vi "Położenie robota z uwzględnieniem jego ewentualnej zmiany.vi"(6 "Boolean in":refnum<vi>, 7 "Parametry robota":T1={"Promień koła [m]"=0.045, "Szerokość robota [m]"=0.37}, 9 "Nowa Odl. od startu[m]":cluster{"X [m]":dbl, "Y [m]":dbl}={"X [m]"=-27.201483053257306, "Y [m]"=-30.40589390754667}, 10 "Azymut robota pocz./nowy":dbl, 11 "Prędkości kół":cluster{"prawe [rad/s]":dbl, "lewe [rad/s]":dbl}) -> (0 "Zmiana położenia robota?":bool, 1 "Azymut [stopnie]":dbl, 2 "Odległość robota od startu":cluster{"X[m]":dbl, "Y[m]":dbl})   [LabVIEW 2012, in "Biblioteka moduł map v3.lvlib" / "Matematyczne.lvlib"]
uses:
  Matematyczne.lvlib
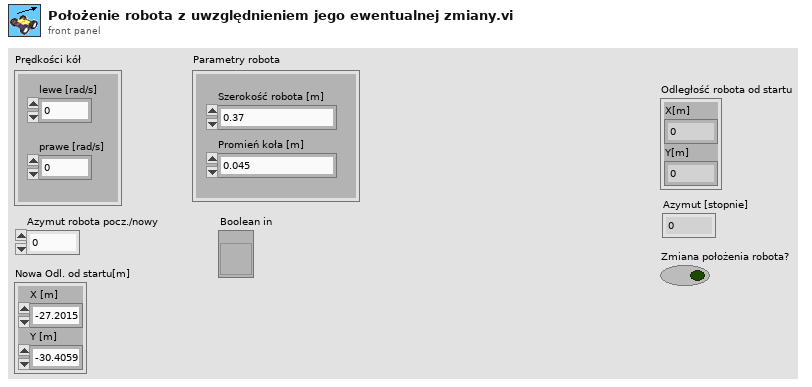
[diagram p1: front panel]
types:
  T1 = cluster{"Promień koła [m]":dbl, "Szerokość robota [m]":dbl}
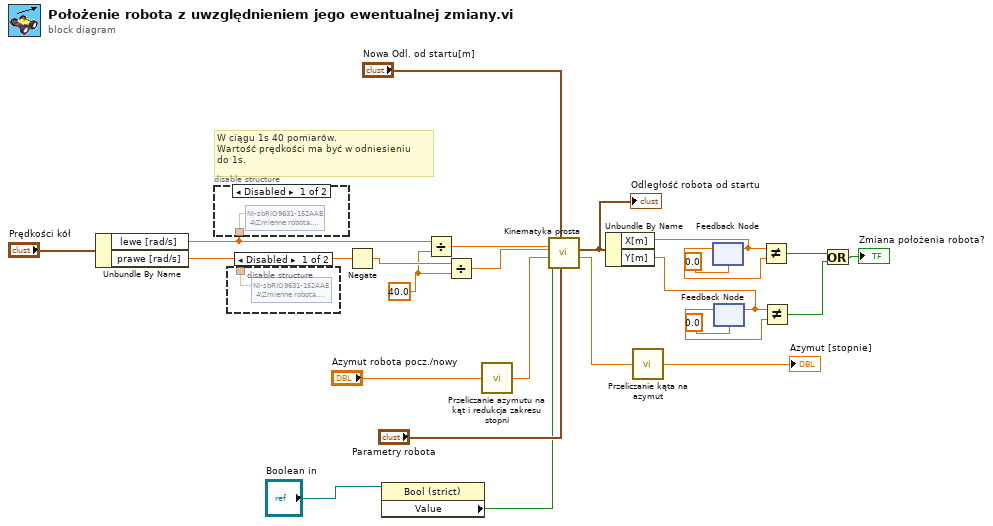
[diagram p0: block diagram]
diagram:
  w4 = 40.0 ("y")
  # "W ciągu 1s 40 pomiarów.\nWartość prędkości ma być w odniesieniu\ndo 1s."
  n1 = Unbundle By Name("Prędkości kół") -> ("lewe [rad/s]"=w8:dbl, "prawe [rad/s]"=w9:dbl)
  n2 = disable-structure shown="Disabled" {
    disable-tunnel: w8 -> [w26 _]
    frame Disabled {
      n3 = shared-variable "NI-sbRIO9631-152AAE4\\Zmienne robota.lvlib\\Vl[rps]"(w26) -> ()  [unwired: 1 in, 1 out]
    }
    frame Enabled {
    }
  }
  n4 = disable-structure shown="Disabled" {
    disable-tunnel: w9 -> [w27 _]
    frame Disabled {
      n5 = shared-variable "NI-sbRIO9631-152AAE4\\Zmienne robota.lvlib\\Vr[rps]"(w27) -> ()  [unwired: 1 in, 1 out]
    }
    frame Enabled {
    }
  }
  n6 = Negate(x=w9) -> (-x=w7:dbl)
  n7 = property class="Bool (strict)"(reference="Boolean in") -> ("Value"=w1:bool)  [unwired: 1 in, 2 out]
  n8 = Divide(x=w8, y=w4) -> (x/y=w6:dbl)
  n9 = Divide(x=w7, y=w4) -> (x/y=w5:dbl)
  n10 = call "Przeliczanie azymutu na kąt i redukcja zakresu stopni.vi"("Azymut [stoponie]"="Azymut robota pocz./nowy") -> ("Kąt [stopnie]"=w22:dbl)  [unwired: 4 in]
  n11 = call "Kinematyka prosta.vi"("Parametry robota"="Parametry robota", "Początkowa odległość robota od startu"="Nowa Odl. od startu[m]", "reset"=w1, "Orientacja pocz./nowa  [stopnie]"=w22, "Prędkość kątowa prawych kół [rad/s]"=w5, "Prędkość kątowa lewych kół [rad/s]"=w6) -> ("Orientacja kąt [stopnie]"=w20:dbl, "Odległość robota od startu"=w11:cluster{"X[m]":dbl, "Y[m]":dbl})  [unwired: 3 in]
  "Odległość robota od startu" <- w11
  n12 = Unbundle By Name(w11) -> ("X[m]"=w15:dbl, "Y[m]"=w14:dbl)
  n13 = call "Przeliczanie kąta na azymut.vi"("Kąt [stoponie]"=w20) -> ("Azymut [stopnie]"=→"Azymut [stopnie]":dbl)  [unwired: 4 in]
  n14 = feedback #1(0.0 ("Y")) -> (w18:dbl)
  n15 = feedback-in #1(w15) -> ()
  n16 = feedback #2(0.0 ("Y")) -> (w16:dbl)
  n17 = feedback-in #2(w14) -> ()
  n18 = Not Equal?(x=w15, y=w18) -> (x != y?=w13:bool)
  n19 = Not Equal?(x=w14, y=w16) -> (x != y?=w12:bool)
  n20 = Or(x=w13, y=w12) -> (x .or. y?=→"Zmiana położenia robota?":bool)
